vi "MFCWrite.vi"(8 "Error In":errorcluster, 11 "Sierra M100 In":refnum<visa-resource-name>) -> (0 "Error Out":errorcluster, 3 "Sierra M100 Out":refnum<visa-resource-name>)   [LabVIEW 2012]
uses:
  MFCConfigurationGlobalAction.ctl
  libs/Sierra-M100/Sierra-M100.lvlib
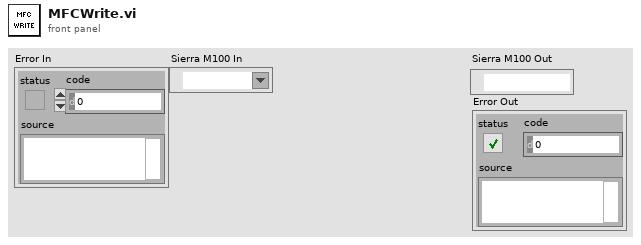
[diagram p1: front panel]
types:
  T1 = typedef "MFCConfigurationGlobalAction.ctl" = enum16{"Get", "Set", "Reset"}
  T2 = typedef "MFCConfiguration.ctl" = cluster{"COM Port":u32, "Timeout (msec)":u32, "Setpoint":dbl, "Valve State":T3, "Gas":T4, "Units":T5, "Serial Number":string, "Firmware Version":string}
  T3 = typedef "Sierra-M100.lvlib/ValveState.ctl" = enum16{"Automatic", "Closed", "Purge"}
  T4 = typedef "Sierra-M100.lvlib/Gas.ctl" = enum16{"Air", "Argon", "CO2", "CO", "Helium", "Hydrogen", "Methane", "Nitrogen", "Nitrous Oxide", "Oxygen"}
  T5 = typedef "Sierra-M100.lvlib/Units.ctl" = enum16{"scc/s", "scc/m", "scc/H", "Ncc/s", "Ncc/m", "Ncc/H", "SCF/s", "SCF/m", "SCF/H", "NM3/s", "NM3/m", "NM3/H", "SM3/s", "SM3/m", "SM3/H", "sl/s", "sl/m", "sl/H", "NL/s", "NL/m", "Nl/H", "g/s", "g/m", "g/H", "kg/s", "kg/m", "kg/H", "lb/s", "lb/m", "lb/H"}
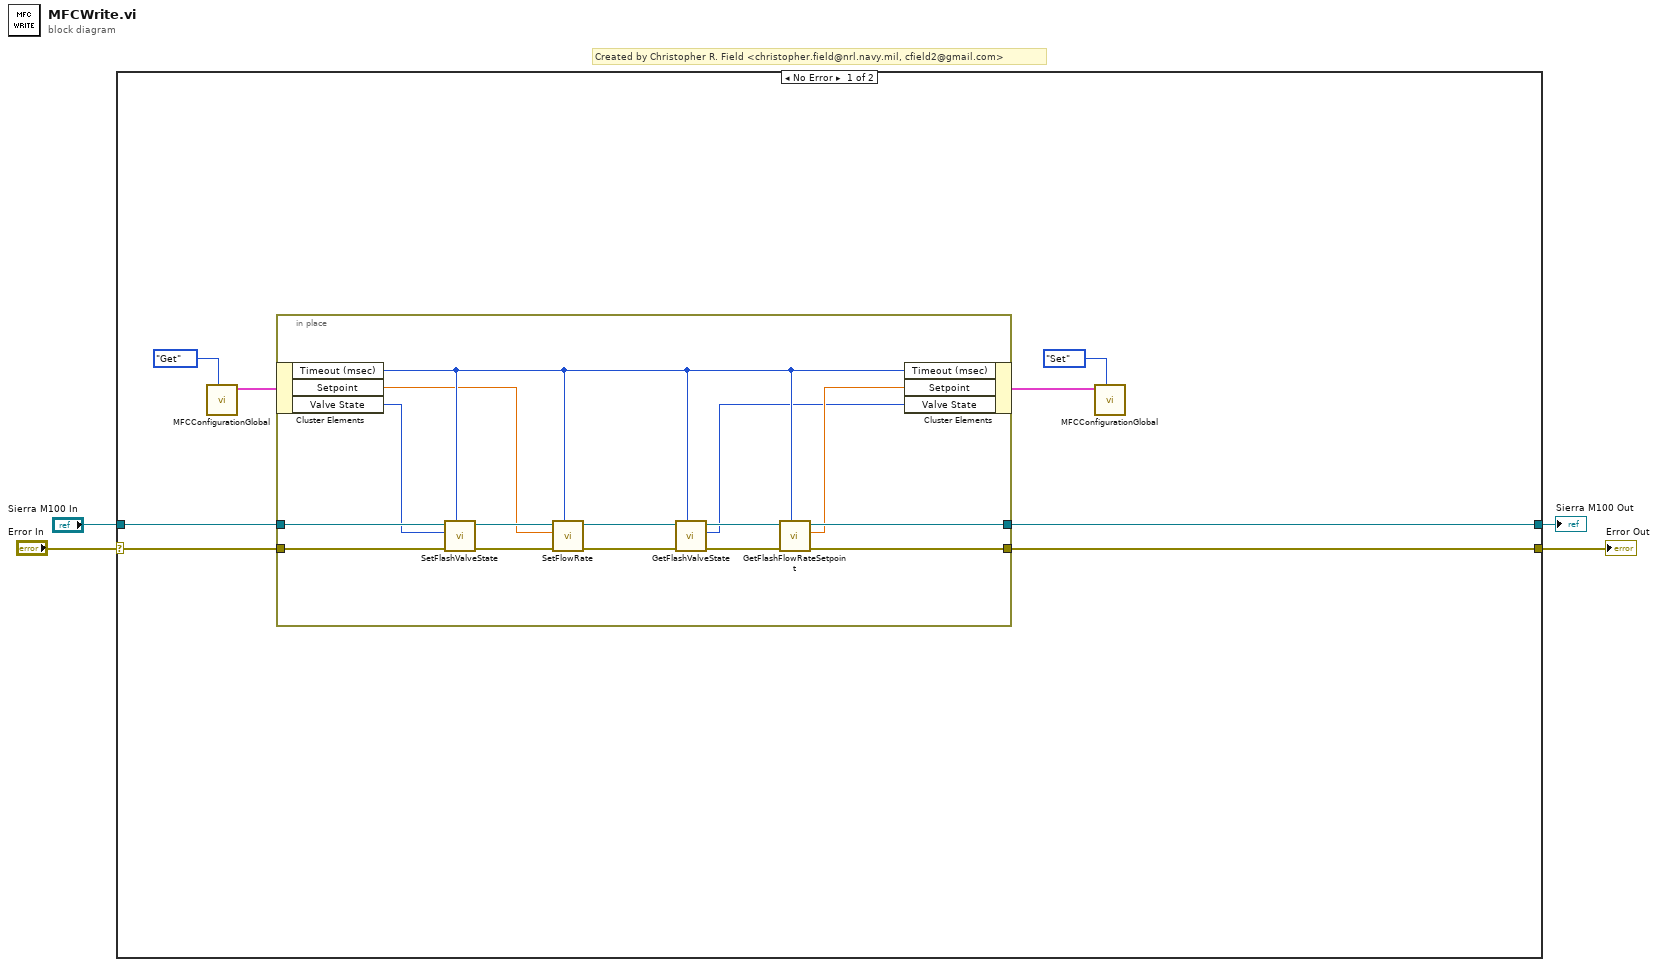
[diagram p0: block diagram]
diagram:
  # "Created by Christopher R. Field <christopher.field@nrl.navy.mil, cfield2@gmail.com>"
  n1 = case shown="No Error" "Error In" {
    selector: "Error In" -> [w12 w28]
    tunnel: "Sierra M100 In" -> [w11 w29]
    tunnel: [w9 w29] -> w2
    tunnel: [w8 w28] -> w1
    frame No Error {
      n2 = call "MFCConfigurationGlobal.vi"("Action"=MFCConfigurationGlobalAction."Get") -> ("Value Out"=w6:T2)  [unwired: 10 in]
      n3 = in-place {
        in-place-border: w12 -> [w27]
        in-place-border: w11 -> [w26]
        in-place-border: [w22] -> w9
        in-place-border: [w21] -> w8
        n4 = in-place-cluster #1(w6) -> ("Timeout (msec)"=w16:u32, "Setpoint"=w13:dbl, "Valve State"=w17:T3)
        n5 = call "SetFlashValveState.vi"("Timeout (ms)"=w16, "Error In"=w27, "Valve State"=w17, "Sierra M100 In"=w26) -> ("Error Out"=w24:errorcluster, "Sierra M100 Out"=w25:refnum<visa-resource-name>)  [unwired: 5 in, 1 out]
        n6 = call "SetFlowRate.vi"("Timeout (ms)"=w16, "Error In"=w24, "Flow Rate (mL/min)"=w13, "Sierra M100 In"=w25) -> ("Error Out"=w20:errorcluster, "Sierra M100 Out"=w23:refnum<visa-resource-name>)  [unwired: 5 in, 1 out]
        n7 = call "GetFlashValveState.vi"("Timeout (ms)"=w16, "Error In"=w20, "Sierra M100 In"=w23) -> ("Error Out"=w18:errorcluster, "Valve State"=w14:T3, "Sierra M100 Out"=w19:refnum<visa-resource-name>)  [unwired: 6 in]
        n8 = call "GetFlashFlowRateSetpoint.vi"("Timeout (ms)"=w16, "Error In"=w18, "Sierra M100 In"=w19) -> ("Error Out"=w21:errorcluster, "Setpoint (mL/min)"=w15:dbl, "Sierra M100 Out"=w22:refnum<visa-resource-name>)  [unwired: 6 in]
        n9 = in-place-cluster #1("Timeout (msec)"=w16, "Setpoint"=w15, "Valve State"=w14) -> (w5:T2)
      }
      n10 = call "MFCConfigurationGlobal.vi"("Action"=MFCConfigurationGlobalAction."Set", "Set Value"=w5) -> ()  [unwired: 9 in, 1 out]
    }
    frame Error {
    }
  }
  "Sierra M100 Out" <- w2
  "Error Out" <- w1
